vi "NISE.local.Get Property DataType.vi"(0 "SLSC Local in":refnum<class "SLSC Interface.lvclass">, 5 "property":refnum<k21>, 11 "error in (no error)":errorcluster) -> (4 "SLSC Local out":refnum<class "SLSC Interface.lvclass">, 6 "property out":refnum<k21>, 10 "Prop.DataType":i32(ring) items=["None", "Bool", "DBL", "I32", "I64", "String", "U32", "U64", "1D Bool", "1D DBL", "1D I32", "1D I64", "1D String", "1D U32", "1D U64"], 15 "error out":errorcluster)   [LabVIEW 2016, in "SLSC Interface.lvclass"]
uses:
  SLSC Interface Class/SLSC Interface.lvclass
  <resource>/objmgr/slsc.rc
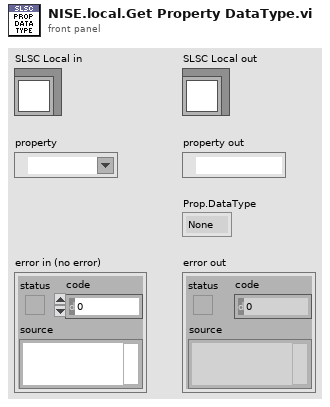
[diagram p1: front panel]
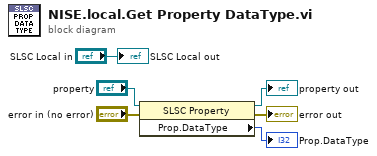
[diagram p0: block diagram]
diagram:
  n1 = property class="SLSC Property"(reference="property", error in="error in (no error)") -> (reference out=→"property out":refnum<k21>, error out=→"error out":errorcluster, "Prop.DataType"=→"Prop.DataType":i32)
  "SLSC Local out" <- "SLSC Local in"
